vi "Store New Connection.vi"(7 "Connection Reference":refnum<data-value>, 8 "error in (no error)":errorcluster, 9 "Active Connection ID":string, 10 "Connection Manager Queue":refnum<class "Message Enqueuer.lvclass">, 11 "MultiplexedConnectionHandler in":refnum<class "MultiplexedConnectionHandler.lvclass">) -> (0 "error out":errorcluster, 3 "MultiplexedConnectionHandler out":refnum<class "MultiplexedConnectionHandler.lvclass">)   [LabVIEW 2019, in "MultiplexedConnectionHandler.lvlib" / "MultiplexedConnectionHandler.lvclass"]
uses:
  <vilib>/gpm_packages/@cs/Network-interface/Source/MultiplexedConnectionHandler/MultiplexedConnectionHandler/MultiplexedConnectionHandler.lvclass
  <vilib>/ActorFramework/Message Enqueuer/Message Enqueuer.lvclass
  <vilib>/gpm_packages/@cs/Network-interface/Source/Connection Reference/Connection Reference/Connection Reference.lvclass
  <vilib>/gpm_packages/@cs/Network-interface/Source/MultiplexedConnectionHandler/MultiplexedConnectionHandler/MultiplexedConnectionHandler.lvclass/MultiplexedConnectionHandler.ctl
  <vilib>/ActorFramework/Message Enqueuer/Message Enqueuer.lvclass/Message Enqueuer.ctl
  <vilib>/ActorFramework/Message Enqueuer/Enqueue.vi
  <vilib>/ActorFramework/Stop Msg/Stop Msg.lvclass
  C:/Program Files/National Instruments/LabVIEW 2019/vi.lib/ActorFramework/Message/Message.lvclass
  <vilib>/ActorFramework/Message Priority Queue/Priority Enqueue.vi
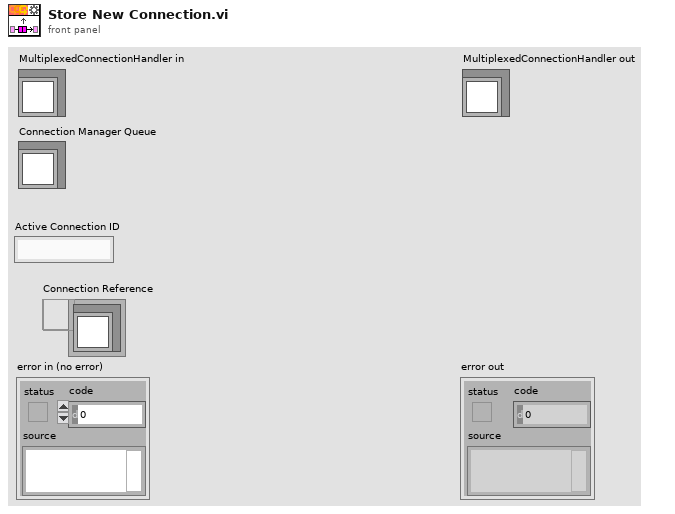
[diagram p1: front panel]
types:
  T1 = cluster{"Connection Manager Queue":refnum<class "Message Enqueuer.lvclass">, "Connection Reference":refnum<data-value>}
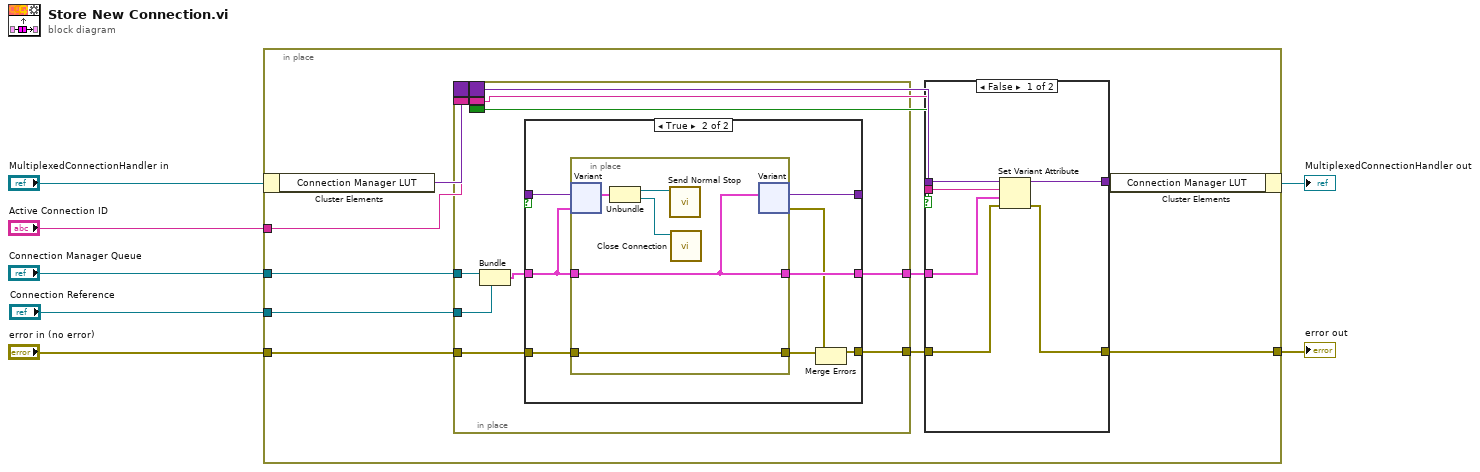
[diagram p0: block diagram]
diagram:
  n1 = in-place {
    in-place-border: "Active Connection ID" -> [w18]
    in-place-border: "Connection Manager Queue" -> [w17]
    in-place-border: "error in (no error)" -> [w16]
    in-place-border: [w9] -> w2
    in-place-border: "Connection Reference" -> [w8]
    n2 = in-place-cluster #1("MultiplexedConnectionHandler in") -> ("Connection Manager LUT"=w19:variant)
    n3 = in-place {
      border: w19 -> [_]
      border: w18 -> [_]
      border: [_] -> w15
      border: [_] -> w14
      border: [_] -> w13
      in-place-border: w17 -> [w21]
      in-place-border: w16 -> [w28]
      in-place-border: [w24] -> w11
      in-place-border: [w23] -> w10
      in-place-border: w8 -> [w22]
      n4 = Bundle("Connection Manager Queue"=w21, "Connection Reference"=w22) -> (w20:T1)  [unwired: 1 in]
      n5 = case shown="True" w25 {
        tunnel: w28 -> [w30 w39]
        tunnel: w27 -> [w31 w38]
        tunnel: [w31 w37] -> w26
        tunnel: [w29 w36] -> w24
        tunnel: [w30 w34] -> w23
        tunnel: w20 -> [w29 w32]
        frame False {
        }
        frame True {
          n6 = in-place {
            in-place-border: w32 -> [w44]
            in-place-border: w39 -> [w43]
            in-place-border: [w44] -> w36
            in-place-border: [w43] -> w35
            n7 = in-place-variant #2(w38, w32) -> (w42:T1)  [unwired: 1 out]
            n8 = Unbundle(w42) -> ("Connection Manager Queue"=w41:refnum<class "Message Enqueuer.lvclass">, "Connection Reference"=w40:refnum<data-value>)
            n9 = call <vilib>:"Send Normal Stop.vi"("Message Enqueuer"=w41) -> ()  [unwired: 10 in, 1 out]
            n10 = call <vilib>:"Close Connection.vi"("Connection Reference In"=w40) -> ()  [unwired: 10 in, 1 out]
            n11 = in-place-variant #2(w44) -> (w37:variant, w33:errorcluster)
          }
          n12 = Merge Errors(w35, w33) -> (w34:errorcluster)
        }
      }
    }
    n13 = case shown="False" w13 {
      tunnel: w15 -> [w50 w52]
      tunnel: w14 -> [w48 _]
      tunnel: [w49 w52] -> w12
      tunnel: w11 -> [w47 _]
      tunnel: w10 -> [w46 w51]
      tunnel: [w45 w51] -> w9
      frame False {
        n14 = Set Variant Attribute(Variant=w50, name=w48, value=w47, error in=w46) -> (Variant out=w49:variant, error out=w45:errorcluster)  [unwired: 1 out]
      }
      frame True {
      }
    }
    n15 = in-place-cluster #1("Connection Manager LUT"=w12) -> (→"MultiplexedConnectionHandler out":refnum<class "MultiplexedConnectionHandler.lvclass">)
  }
  "error out" <- w2
